vi "PH_Stepmotor_BaseClass.Axis DIM get Tagname.vi"(1 "Tag":T1, 2 "Instancename":T2={"Instance"="N/A", "Motor Nr"=0}) -> (0 "Axis Tagname":string)   [LabVIEW 2014, in "PH_Stepmotor_BaseClass.lvlib"]
doc: "This VI concatenates a Tagname out of a strict type def enum control and other information. It keeps also the information whether the Tag is existing (if not, N/A is given out as name)."
uses:
  PH_Stepmotor_BaseClass.lvlib
  PH_Stepmotor_BaseClass.Axis Address.ctl
  PH_Stepmotor_BaseClass.Axis DIM Tags.ctl
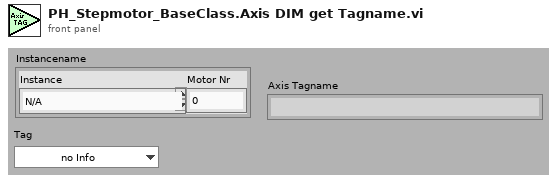
[diagram p1: front panel]
types:
  T1 = typedef "PH_Stepmotor_BaseClass.lvlib/PH_Stepmotor_BaseClass.Axis DIM Tags.ctl" = enum16{"no Info", "Information", "Settings"}
  T2 = typedef "PH_Stepmotor_BaseClass.lvlib/PH_Stepmotor_BaseClass.Axis Address.ctl" = cluster{"Instance":string, "Motor Nr":i32}
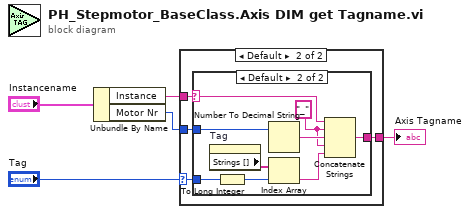
[diagram p0: block diagram]
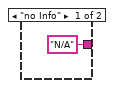
[diagram p2: hidden frame]
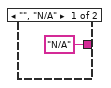
[diagram p3: hidden frame]
diagram:
  n1 = Unbundle By Name("Instancename") -> ("Instance"=w2:string, "Motor Nr"=w1:i32)
  n2 = case shown="Default" "Tag" {
    selector: "Tag" -> [_ w7]
    tunnel: w1 -> [_ w10]
    tunnel: ["N/A" w9] -> w5
    tunnel: w2 -> [_ w8]
    frame "no Info" {
    }
    frame Default {
      n3 = case shown="Default" w8 {
        selector: w8 -> [_ w14]
        tunnel: w10 -> [_ w20]
        tunnel: ["N/A" w18] -> w9
        tunnel: w7 -> [_ w13]
        frame "", "N/A" {
        }
        frame Default {
          w17 = "_" ("string")
          n4 = property on="Tag" class="Enum (strict)"() -> ("Strings []"=w16:string[])  [unwired: 2 in, 2 out]
          n5 = To Long Integer(number=w13) -> (32bit integer=w12:i32)
          n6 = Number To Decimal String(number=w20) -> (decimal integer string=w19:string)  [unwired: 1 in]
          n7 = Index Array(array=w16, index=w12) -> (element=w15:string)
          n8 = Concatenate Strings(w14, w17, w19, w17, w15) -> (w18:string)
        }
      }
    }
  }
  "Axis Tagname" <- w5
